vi "Resulting resolution.vi"(1 "AO.Resolution":dbl, 2 "Supported AO voltage ranges":dbl[](array[numeric]) format="%#.2f", 3 "Lower voltage limit (V)":dbl format="%.6f", 4 "Upper voltage limit (V)":dbl=10.0 format="%.6f", 5 "error in":errorcluster) -> (10 "Res. AO.Resolution G0":dbl, 12 "Vmin G0":dbl format="%#.2f", 13 "Vmax G0":dbl format="%#_2g", 14 "Vmin":dbl format="%#.2f", 15 "Vmax":dbl format="%#_2g", 16 "Gain":dbl format="%#_2g", 17 "Res. AO.Resolution":dbl, 19 "error out":errorcluster)   [LabVIEW 2026]
doc: "This vi calculates which analog output voltage range is best for the given Lower and Upper voltage limit and returns the appropriate offset and the resulting resolution value. It does also calculate range and resolution if gain must be zero.\n\nValid for Analog systems."
panel:
  # "This vi calculates which analog output voltage range is best for the given Lower and Upper voltage limit and returns the appropriate \noffset and the resulting resolution value. It does also calculate range and resolution if gain must be zero."
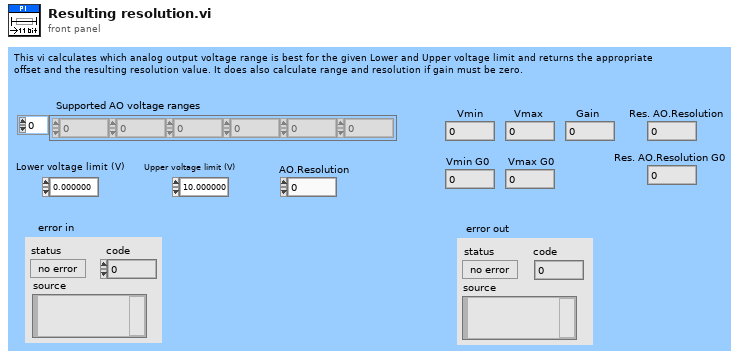
[diagram p1: front panel]
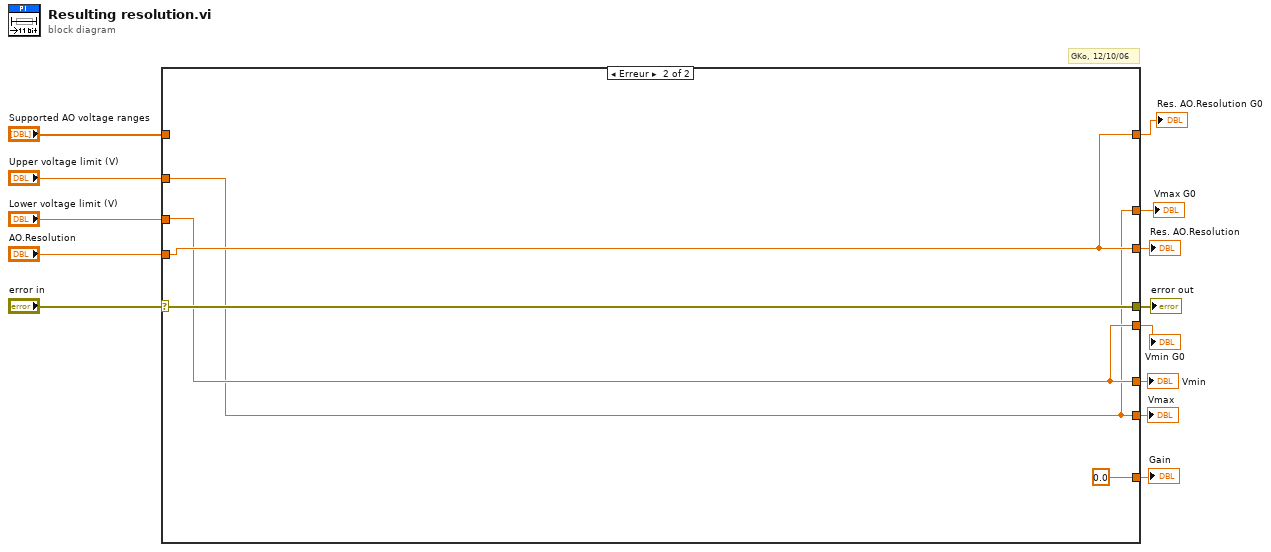
[diagram p0: block diagram]
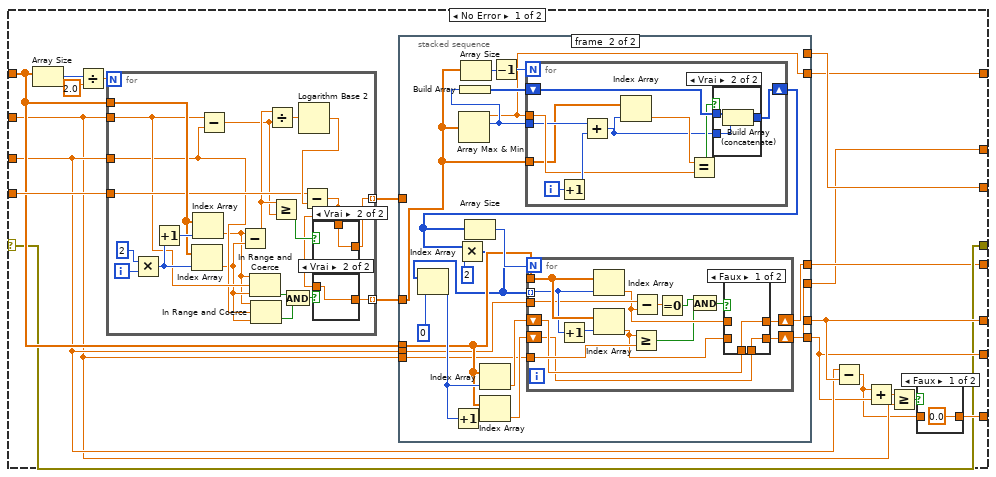
[diagram p2: hidden frame]
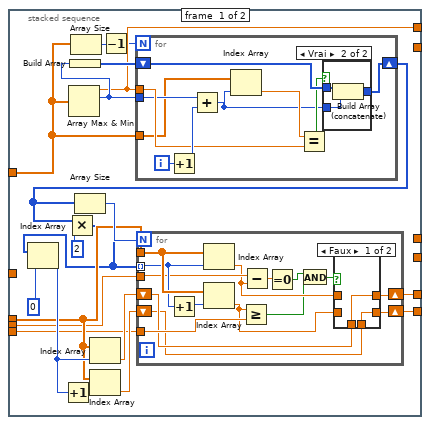
[diagram p3: hidden frame]
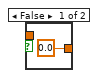
[diagram p9: hidden frame]
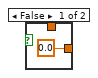
[diagram p10: hidden frame]
diagram:
  # "GKo, 12/10/06"
  n1 = case shown="Erreur" "error in" {
    selector: "error in" -> [w19 w171]
    tunnel: [w19 w171] -> w12
    tunnel: "Supported AO voltage ranges" -> [w28 _]
    tunnel: "Lower voltage limit (V)" -> [w26 w168]
    tunnel: "Upper voltage limit (V)" -> [w23 w167]
    tunnel: "AO.Resolution" -> [w30 w169]
    tunnel: [w29 w169] -> w7
    tunnel: [w27 w168] -> w6
    tunnel: [w25 w167] -> w5
    tunnel: [w20 0.0] -> w4
    tunnel: [w16 w169] -> w3
    tunnel: [w15 w168] -> w2
    tunnel: [w14 w167] -> w1
    frame No Error {
      n2 = Array Size(array=w28) -> (size(s)=w33:i32)
      n3 = Divide(x=w33, y=2.0) -> (x/y=w31:dbl)
      n4 = for {
        N: w31 -> [_]
        tunnel: w26 -> [w149]
        tunnel: w28 -> [w159]
        tunnel: w30 -> [w158]
        tunnel: w23 -> [w150]
        tunnel: [w151] -> w18 mode=indexing
        tunnel: [w142] -> w17 mode=indexing
        i -> [w157]
        n5 = Multiply(x=2, y=w157) -> (x*y=w155:i32)
        n6 = Increment(x=w155) -> (x+1=w160:i32)
        n7 = Index Array(array=w159, index=w155) -> (element=w148:dbl)
        n8 = Index Array(array=w159, index=w160) -> (element=w147:dbl)
        n9 = Subtract(x=w150, y=w149) -> (x-y=w153:dbl)
        n10 = Subtract(x=w147, y=w148) -> (x-y=w154:dbl)
        n11 = In Range and Coerce(upper limit=w147, x=w150, lower limit=w148) -> (In Range?=w145:bool)  [unwired: 1 out]
        n12 = In Range and Coerce(upper limit=w147, x=w149, lower limit=w148) -> (In Range?=w144:bool)  [unwired: 1 out]
        n13 = Divide(x=w154, y=w153) -> (x/y=w162:dbl)
        n14 = Greater Or Equal?(x=w154, y=w153) -> (x >= y?=w152:bool)
        n15 = And(x=w145, y=w144) -> (x .and. y?=w146:bool)
        n16 = Logarithm Base 2(1:w162) -> (0:w161:dbl)
        n17 = Subtract(x=w158, y=w161) -> (x-y=w143:dbl)
        n18 = case shown="Vrai" w152 {
          tunnel: [0.0 w166] -> w151
          tunnel: w143 -> [_ w166]
          frame False {
          }
          frame True {
          }
        }
        n19 = case shown="Vrai" w146 {
          tunnel: [0.0 w164] -> w142
          tunnel: w143 -> [_ w164]
          frame False {
          }
          frame True {
          }
        }
      }
      n20 = stacked-sequence {
        tunnel: [w51 _] -> w29
        tunnel: w28 -> [w44 w98]
        tunnel: [w43 _] -> w27
        tunnel: w26 -> [w42 w97]
        tunnel: [w41 _] -> w25
        tunnel: w23 -> [w40 w96]
        tunnel: w18 -> [w39 _]
        tunnel: w17 -> [_ w90]
        tunnel: [_ w89] -> w16
        tunnel: [_ w88] -> w15
        tunnel: [_ w87] -> w14
        frame #0 {
          n21 = Array Max & Min(array=w39) -> (max value=w51:dbl, max index (indices)=w53:i32)  [unwired: 2 out]
          n22 = Build Array(w53) -> (w52:i32[])
          n23 = Array Size(array=w39) -> (size(s)=w38:i32)
          n24 = Decrement(x=w38) -> (x-1=w37:i32)
          n25 = for {
            N: w37 -> [_]
            tunnel: w39 -> [w56]
            tunnel: w53 -> [w60]
            tunnel: w51 -> [w61]
            shift-right: [w59] -> w36
            shift-left: w52 -> [w58]
            i -> [w63]
            n26 = Increment(x=w63) -> (x+1=w62:i32)
            n27 = Add(x=w60, y=w62) -> (x+y=w54:i32)
            n28 = Index Array(array=w56, index=w54) -> (element=w55:dbl)
            n29 = Equal?(x=w55, y=w61) -> (x = y?=w57:bool)
            n30 = case shown="Vrai" w57 {
              tunnel: w58 -> [w64 w67]
              tunnel: w54 -> [_ w65]
              tunnel: [w64 w66] -> w59
              frame False {
              }
              frame True {
                n31 = Build Array (concatenate)(w67, w65) -> (w66:i32[])
              }
            }
          }
          n32 = Multiply(x=w36, y=2) -> (x*y=w34:i32[])
          n33 = Index Array(array=w34, index=0) -> (element=w48:i32)
          n34 = Increment(x=w48) -> (x+1=w47:i32)
          n35 = Array Size(array=w36) -> (size(s)=w50:i32)
          n36 = Index Array(array=w44, index=w48) -> (element=w46:dbl)
          n37 = Index Array(array=w44, index=w47) -> (element=w45:dbl)
          n38 = for {
            N: w50 -> [_]
            tunnel: w44 -> [w82]
            tunnel: w34 -> [w80] mode=indexing
            tunnel: w42 -> [w79]
            tunnel: w40 -> [w75]
            shift-right: [w72] -> w43
            shift-left: w46 -> [w69]
            shift-right: [w70] -> w41
            shift-left: w45 -> [w68]
            n39 = Increment(x=w80) -> (x+1=w81:i32)
            n40 = Index Array(array=w82, index=w80) -> (element=w77:dbl)
            n41 = Index Array(array=w82, index=w81) -> (element=w71:dbl)
            n42 = Greater Or Equal?(x=w71, y=w75) -> (x >= y?=w74:bool)
            n43 = Subtract(x=w79, y=w77) -> (x-y=w78:dbl)
            n44 = Equal To 0?(x=w78) -> (x = 0?=w76:bool)
            n45 = And(x=w76, y=w74) -> (x .and. y?=w73:bool)
            n46 = case shown="Faux" w73 {
              tunnel: w77 -> [_ w86]
              tunnel: [w84 w86] -> w72
              tunnel: w71 -> [_ w85]
              tunnel: [w83 w85] -> w70
              tunnel: w69 -> [w84 _]
              tunnel: w68 -> [w83 _]
              frame False {
              }
              frame True {
              }
            }
          }
        }
        frame #1 {
          n47 = Array Max & Min(array=w90) -> (max value=w89:dbl, max index (indices)=w106:i32)  [unwired: 2 out]
          n48 = Build Array(w106) -> (w105:i32[])
          n49 = Array Size(array=w90) -> (size(s)=w95:i32)
          n50 = Decrement(x=w95) -> (x-1=w94:i32)
          n51 = for {
            N: w94 -> [_]
            tunnel: w90 -> [w109]
            tunnel: w106 -> [w113]
            tunnel: w89 -> [w114]
            shift-right: [w112] -> w93
            shift-left: w105 -> [w111]
            i -> [w116]
            n52 = Increment(x=w116) -> (x+1=w115:i32)
            n53 = Add(x=w113, y=w115) -> (x+y=w107:i32)
            n54 = Index Array(array=w109, index=w107) -> (element=w108:dbl)
            n55 = Equal?(x=w108, y=w114) -> (x = y?=w110:bool)
            n56 = case shown="Vrai" w110 {
              tunnel: w111 -> [w117 w120]
              tunnel: w107 -> [_ w118]
              tunnel: [w117 w119] -> w112
              frame False {
              }
              frame True {
                n57 = Build Array (concatenate)(w120, w118) -> (w119:i32[])
              }
            }
          }
          n58 = Multiply(x=w93, y=2) -> (x*y=w91:i32[])
          n59 = Index Array(array=w91, index=0) -> (element=w102:i32)
          n60 = Increment(x=w102) -> (x+1=w101:i32)
          n61 = Array Size(array=w93) -> (size(s)=w104:i32)
          n62 = Index Array(array=w98, index=w102) -> (element=w100:dbl)
          n63 = Index Array(array=w98, index=w101) -> (element=w99:dbl)
          n64 = for {
            N: w104 -> [_]
            tunnel: w98 -> [w135]
            tunnel: w91 -> [w133] mode=indexing
            tunnel: w97 -> [w132]
            tunnel: w96 -> [w128]
            shift-right: [w125] -> w88
            shift-left: w100 -> [w122]
            shift-right: [w123] -> w87
            shift-left: w99 -> [w121]
            n65 = Increment(x=w133) -> (x+1=w134:i32)
            n66 = Index Array(array=w135, index=w133) -> (element=w130:dbl)
            n67 = Index Array(array=w135, index=w134) -> (element=w124:dbl)
            n68 = Greater Or Equal?(x=w124, y=w128) -> (x >= y?=w127:bool)
            n69 = Subtract(x=w132, y=w130) -> (x-y=w131:dbl)
            n70 = Equal To 0?(x=w131) -> (x = 0?=w129:bool)
            n71 = And(x=w129, y=w127) -> (x .and. y?=w126:bool)
            n72 = case shown="Faux" w126 {
              tunnel: w130 -> [_ w139]
              tunnel: [w137 w139] -> w125
              tunnel: w124 -> [_ w138]
              tunnel: [w136 w138] -> w123
              tunnel: w122 -> [w137 _]
              tunnel: w121 -> [w136 _]
              frame False {
              }
              frame True {
              }
            }
          }
        }
      }
      n73 = Subtract(x=w26, y=w27) -> (x-y=w21:dbl)
      n74 = Add(x=w21, y=w25) -> (x+y=w24:dbl)
      n75 = Greater Or Equal?(x=w24, y=w23) -> (x >= y?=w22:bool)
      n76 = case shown="Faux" w22 {
        tunnel: w21 -> [_ w141]
        tunnel: [0.0 w141] -> w20
        frame False {
        }
        frame True {
        }
      }
    }
    frame Error {
    }
  }
  "error out" <- w12
  "Res. AO.Resolution" <- w7
  "Gain" <- w4
  "Vmin" <- w6
  "Vmax" <- w5
  "Vmin G0" <- w2
  "Vmax G0" <- w1
  "Res. AO.Resolution G0" <- w3
